vi "tabulateData.vi"(8 "error in (no error)":errorcluster, 11 "RfOutputData in":refnum<class "RfOutputData.lvclass">) -> (0 "error out":errorcluster, 3 "RfOutputData out":refnum<class "RfOutputData.lvclass">)   [LabVIEW 2009, in "DataMappers.lvlib" / "RfOutputData.lvclass"]
uses:
  RfOutputData.lvclass
  DatabaseHelpers/Database Objects/Channel/RfOutputChannel/RfOutputChannel.lvclass
panel:
  in  "Array":T1(array[cluster])
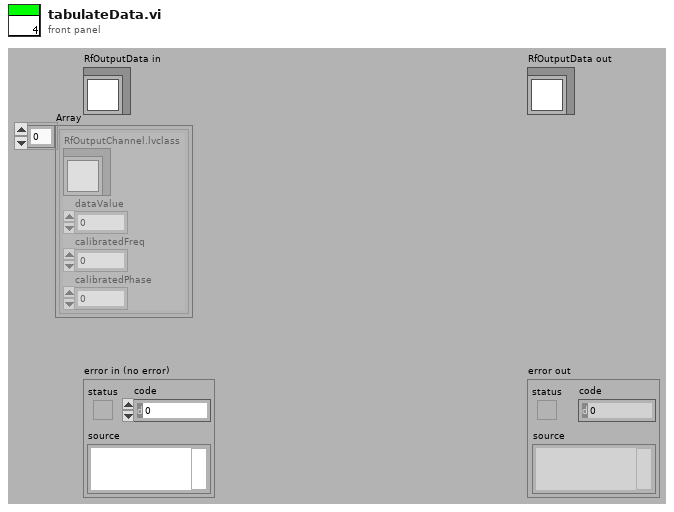
[diagram p1: front panel]
types:
  T1 = cluster{"RfOutputChannel.lvclass":refnum<class "RfOutputChannel.lvclass">, "dataValue":dbl, "calibratedFreq":dbl, "calibratedPhase":dbl}[]
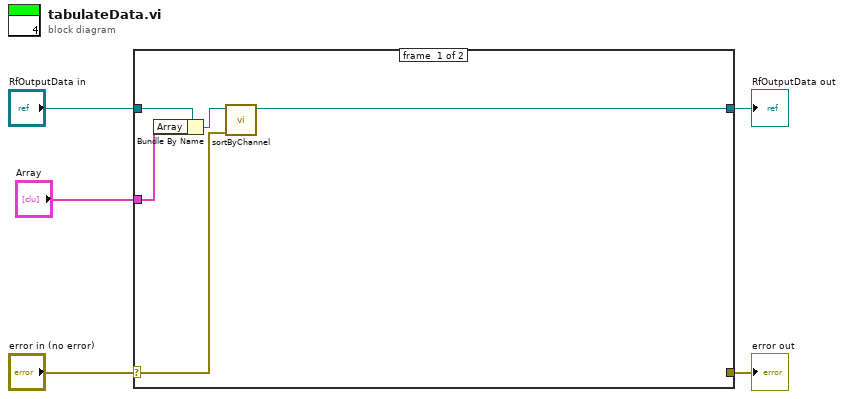
[diagram p0: block diagram]
diagram:
  n1 = case shown="No Error" "error in (no error)" {
    selector: "error in (no error)" -> [w6 w12]
    tunnel: [_ w12] -> w4
    tunnel: [w7 w11] -> w2
    tunnel: "RfOutputData in" -> [w9 w11]
    tunnel: "Array" -> [w10 _]
    frame #0 {
      n2 = Bundle By Name(cluster=w9, "Array"=w10) -> (w8:refnum<class "RfOutputData.lvclass">)
      n3 = call "sortByChannel.vi"("error in (no error)"=w6, "RfOutputData in"=w8) -> ("RfOutputData out"=w7:refnum<class "RfOutputData.lvclass">)  [unwired: 7 in, 2 out]
    }
    frame #1 {
    }
  }
  "error out" <- w4
  "RfOutputData out" <- w2
